vi "SAVE IN DB.vi"(8 "error in (no error)":errorcluster, 10 "SAVE IN DB Argument":cluster{"MONEY":T1, "PRODUCTS":T2, "DB?":bool} {"MONEY"."MONEY" format="%#_3g"}) -> (0 "error out":errorcluster)   [LabVIEW 2019, in "CONFIGURATION.lvlib"]
doc: "HERE WE CAN SAVE NEW COINS AND VALUES \n_____\nCreated using Delacor QMH Event Scripter 5.0.0.112."
uses:
  CONFIGURATION.lvlib
  DB_VENDING MACHINE/Type Defs/MONEY.ctl
  DB_VENDING MACHINE/Type Defs/PRODUCTS.ctl
  SAVE IN DB Argument--cluster.ctl
  DB_VENDING MACHINE/DB_VENDING MACHINE.lvlib
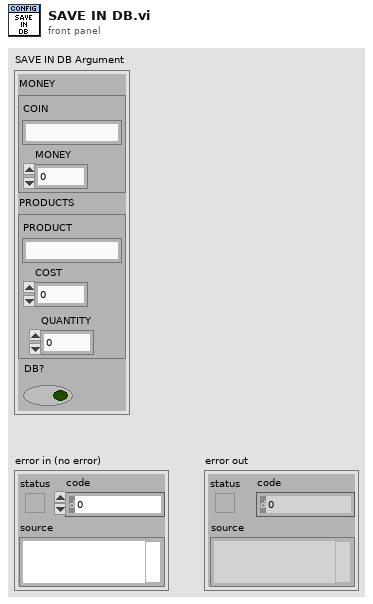
[diagram p1: front panel]
types:
  T1 = typedef "DB_VENDING MACHINE.lvlib/MONEY.ctl" = cluster{"COIN":string, "MONEY":dbl}
  T2 = typedef "DB_VENDING MACHINE.lvlib/PRODUCTS.ctl" = cluster{"PRODUCT":string, "COST":dbl, "QUANTITY":i8}
  T3 = typedef "CONFIGURATION.lvlib/SAVE IN DB Argument--cluster.ctl" = cluster{"MONEY":T1, "PRODUCTS":T2, "DB?":bool}
  T4 = typedef "CONFIGURATION.lvlib/Request Events--cluster.ctl" = cluster{"Stop Module":refnum<user-event>, "Show Panel":refnum<user-event>, "Hide Panel":refnum<user-event>, "Get Module Execution Status":refnum<user-event>, "Show Diagram":refnum<user-event>, "SET CONFIGURATIO":refnum<user-event>, "UPDATE DB TO MONEY LIST":refnum<user-event>, "SAVE IN DB":refnum<user-event>, "SAVE PRODUCT IN DATABASE":refnum<user-event>, "UPDATE DB TO PRODUCT LIST":refnum<user-event>}
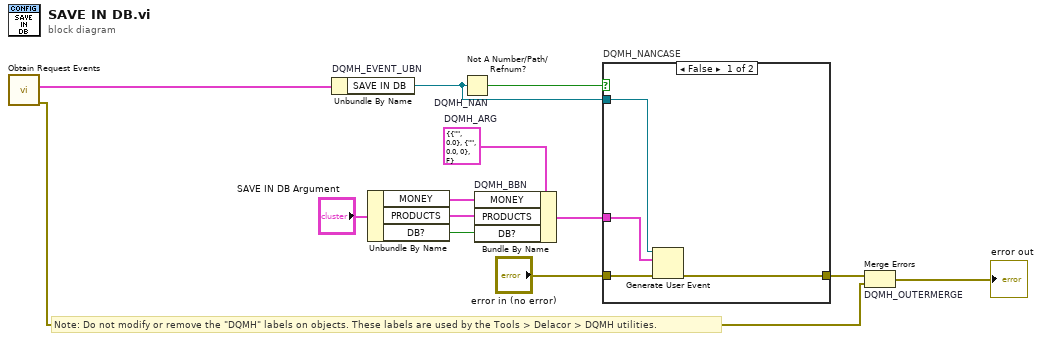
[diagram p0: block diagram]
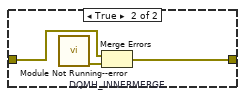
[diagram p2: hidden frame]
diagram:
  w7 = T3 {"MONEY"={"COIN"="", "MONEY"=0.0}, "PRODUCTS"={"PRODUCT"="", "COST"=0.0, "QUANTITY"=0}, "DB?"=FALSE}  # DQMH_ARG
  # "Note: Do not modify or remove the \"DQMH\" labels on objects. These labels are used by the Tools > Delacor > DQMH utilities."
  n1 = call "Obtain Request Events.vi"() -> ("error out"=w6:errorcluster, "CONFIGURATION Request Events"=w5:T4)  [unwired: 10 in]
  n2 = Unbundle By Name "DQMH_EVENT_UBN"(w5) -> ("SAVE IN DB"=w9:refnum<user-event>)
  n3 = Unbundle By Name("SAVE IN DB Argument") -> ("MONEY"=w3:T1, "PRODUCTS"=w2:T2, "DB?"=w1:bool)
  n4 = Not A Number/Path/Refnum? "DQMH_NAN"(number/path/refnum=w9) -> (NaN/Path/Refnum?=w10:bool)
  n5 = Bundle By Name "DQMH_BBN"(cluster=w7, "MONEY"=w3, "PRODUCTS"=w2, "DB?"=w1) -> (w11:T3)
  n6 = case "DQMH_NANCASE" shown="False" w10 {
    tunnel: "error in (no error)" -> [w17 w20]
    tunnel: [w16 w19] -> w8
    tunnel: w9 -> [w15 _]
    tunnel: w11 -> [w14 _]
    frame False {
      n7 = Generate User Event(user event=w15, event data cluster=w14, error in=w17) -> (error out=w16:errorcluster)  [unwired: 1 in, 1 out]
    }
    frame True {
      n8 = call "Module Not Running--error.vi"() -> ("error out"=w18:errorcluster)  [unwired: 11 in]
      n9 = Merge Errors "DQMH_INNERMERGE"(w20, w18) -> (w19:errorcluster)
    }
  }
  n10 = Merge Errors "DQMH_OUTERMERGE"(w8, w6) -> (→"error out":errorcluster)
